vi "16 to 10.vi"(10 "字符串":string) -> (2 "字符串 2":string)   [LabVIEW 2021]
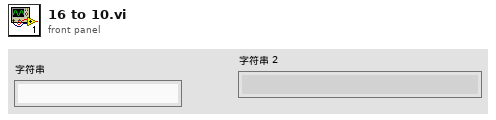
[diagram p1: front panel]
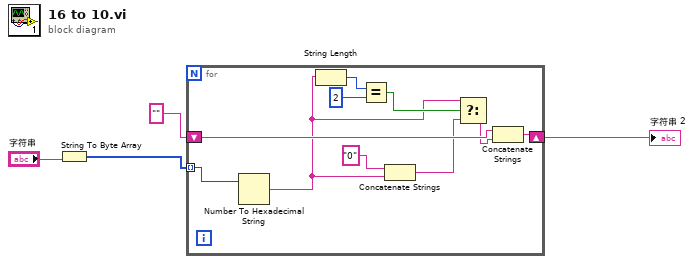
[diagram p0: block diagram]
diagram:
  n1 = String To Byte Array(string="字符串") -> (unsigned byte array=w1:u8[])
  n2 = for {
    shift-right: [w13] -> w3
    shift-left: "" -> [w14]
    tunnel: w1 -> [w12] mode=indexing
    n3 = Number To Hexadecimal String(2:w12) -> (0:w8:string)  [unwired: 1 in]
    n4 = String Length(string=w8) -> (length=w11:i32)
    n5 = Equal?(x=w11, y=2) -> (x = y?=w9:bool)
    n6 = Concatenate Strings("0", w8) -> (w6:string)
    n7 = Select(t=w8, s=w9, f=w6) -> (s? t:f=w5:string)
    n8 = Concatenate Strings(w14, w5) -> (w13:string)
  }
  "字符串 2" <- w3
